vi "basehorno.vi"() -> ()   [LabVIEW 2017]
panel:
  out "Numeric 2":dbl
  out "Boolean 3":bool
  out "Numeric":dbl
  out "Boolean 4":bool
  in  "Boolean 2":bool
  out "Tank":dbl(slide) scale=0.0..100.0
  out "Valvula gas":bool
  out "Valvula aire":bool
  out "Slide 5":dbl(slide) scale=0.0..10.0
  out "Slide 4":dbl(slide) scale=0.0..10.0
  out "Slide 3":dbl(slide) scale=0.0..10.0
  out "HORNO":bool
  out "Slide 2":dbl(slide) scale=0.0..10.0
  in  "stop":bool
  in  "inicio":bool
  out "GAS":bool
  out "AIRE":bool
  # "INTEGRANTES:\nMARIA JOSE CORTEZ H.\nGROVER ARUQUIPA"
  # "PROCESO SIDERURGICO DE FUNDICION"
  # "COQUE"
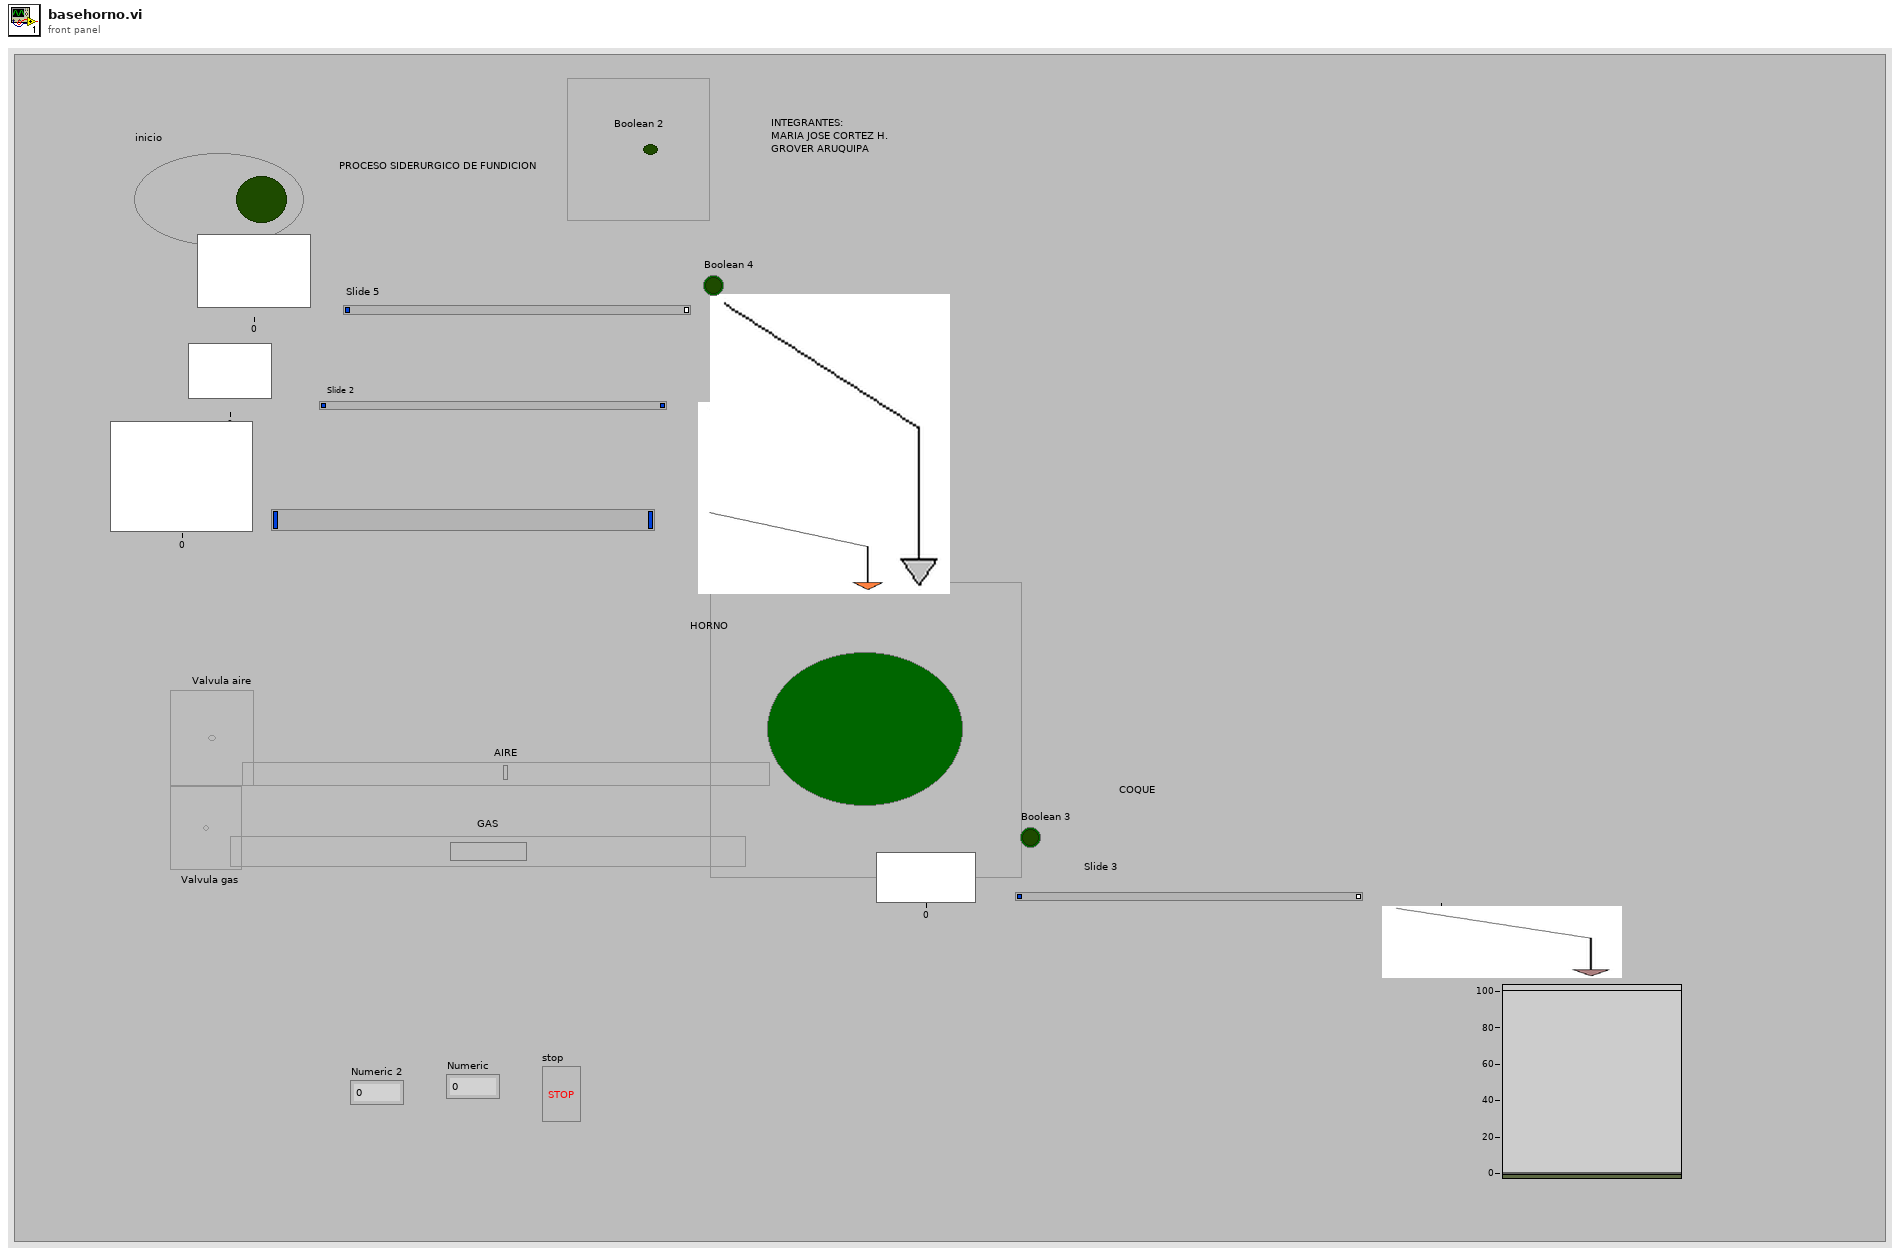
[diagram p1: front panel]
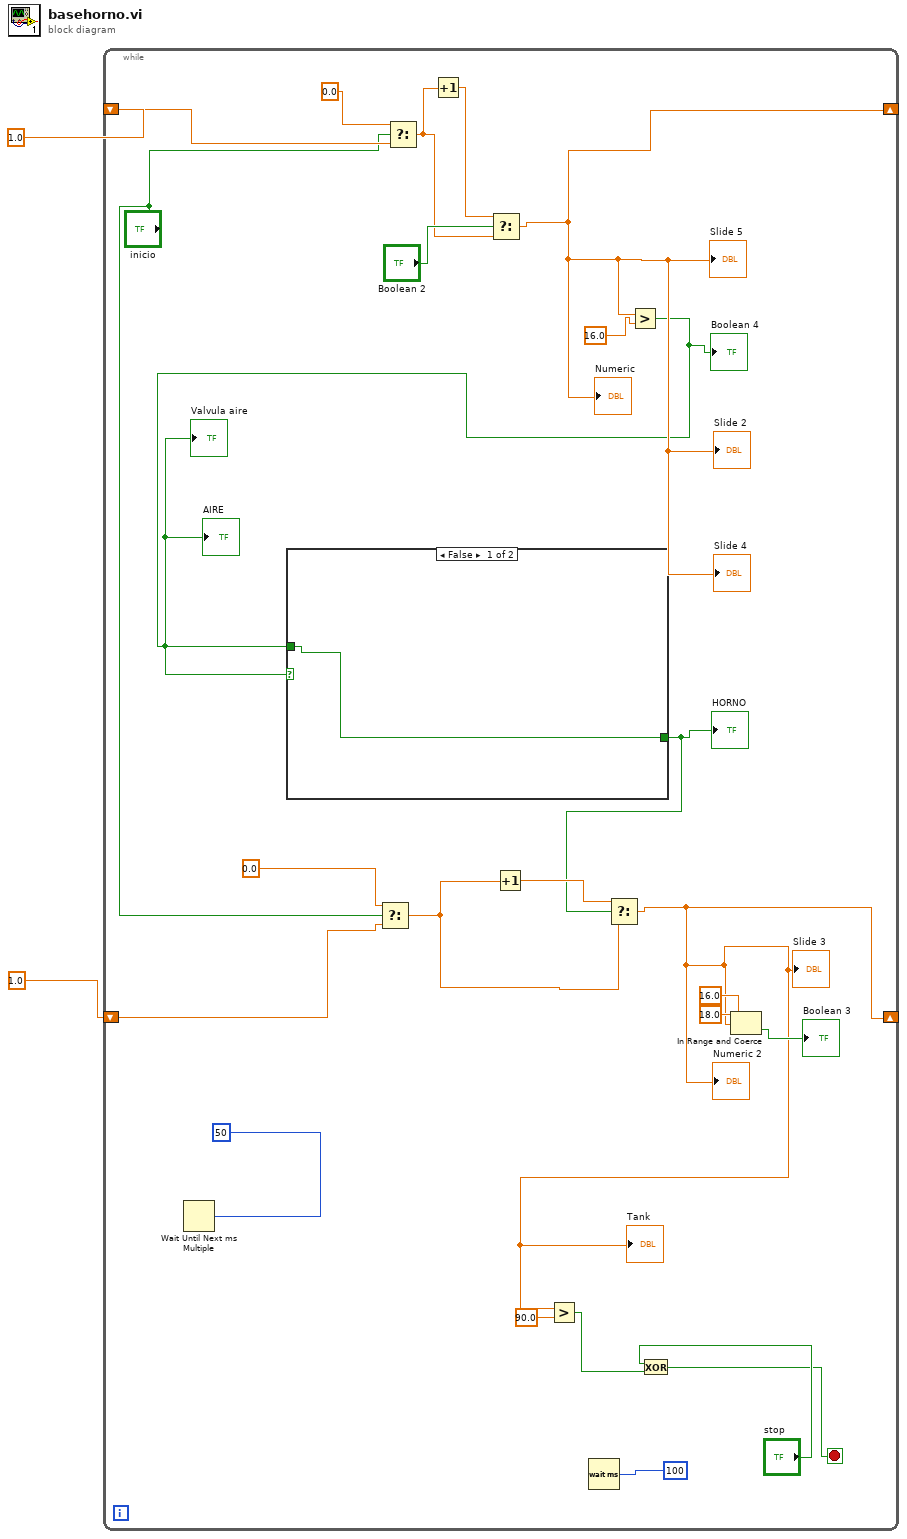
[diagram p0: block diagram]
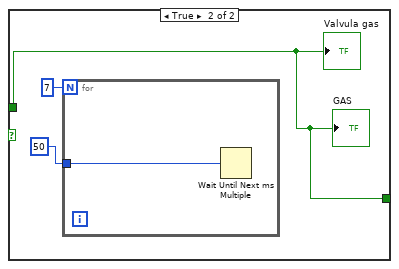
[diagram p2: hidden frame]
diagram:
  n1 = while {
    shift-right: [w20] -> _
    shift-left: 1.0 ("t") -> [w24]
    shift-right: [w7] -> _
    shift-left: 1.0 ("t") -> [w10]
    stop <- w3 stop-if-true
    n2 = Wait Until Next ms Multiple(millisecond multiple=u32 50) -> ()  [unwired: 1 out]
    n3 = Select(t=0.0, s="inicio", f=w10) -> (s? t:f=w15:dbl)
    n4 = Select(t=0.0 ("f"), s="inicio", f=w24) -> (s? t:f=w21:dbl)
    n5 = Increment(x=w21) -> (x+1=w23:dbl)
    n6 = Select(t=w23, s="Boolean 2", f=w21) -> (s? t:f=w20:dbl)
    "Slide 2" <- w20
    "Slide 4" <- w20
    "Slide 5" <- w20
    "Numeric" <- w20
    n7 = Increment(x=w15) -> (x+1=w16:dbl)
    n8 = Wait (ms)(milliseconds to wait=u32 100) -> ()  [unwired: 1 out]
    n9 = Greater?(x=w20, y=16.0 ("lower limit")) -> (0:w18:bool)
    "AIRE" <- w18
    "Valvula aire" <- w18
    "Boolean 4" <- w18
    n10 = case shown="False" w18 {
      tunnel: w18 -> [w27 w28]
      tunnel: [w27 w28] -> w9
      frame False {
      }
      frame True {
        n11 = for {
          N: 7 -> [_]
          tunnel: u32 50 ("millisecond multiple") -> [w31]
          n12 = Wait Until Next ms Multiple(millisecond multiple=w31) -> ()  [unwired: 1 out]
        }
        "Valvula gas" <- w28
        "GAS" <- w28
      }
    }
    "HORNO" <- w9
    n13 = Select(t=w16, s=w9, f=w15) -> (s? t:f=w7:dbl)
    "Slide 3" <- w7
    "Numeric 2" <- w7
    "Tank" <- w7
    n14 = Greater?(x=w7, y=90.0) -> (0:w4:bool)
    n15 = Exclusive Or(1:w4, 2:"stop") -> (0:w3:bool)
    n16 = In Range and Coerce(upper limit=18.0, x=w7, lower limit=16.0) -> (In Range?=→"Boolean 3":bool)  [unwired: 1 out]
  }
